vi "user32_SendMessage.vi"(5 "IParam":u32, 7 "wParam":u32, 8 "错误输入（无错误）":errorcluster, 9 "Msg":u32, 10 "hWnd":u32, 11 "路径输入":path) -> (0 "错误输出":errorcluster, 3 "返回值":u32)   [LabVIEW 2017]
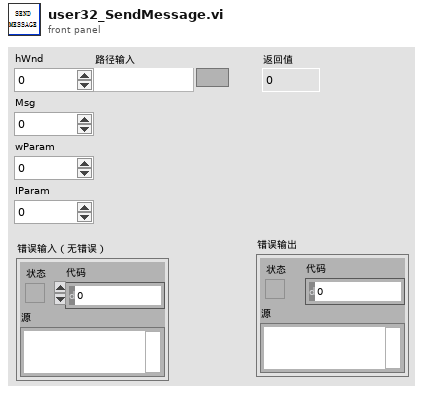
[diagram p1: front panel]
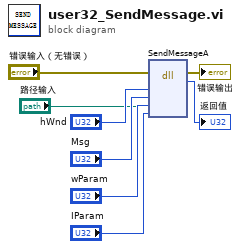
[diagram p0: block diagram]
diagram:
  n1 = dll-call lib="C:/Windows/System32/user32.dll" fn="SendMessageA"(path in="路径输入", error in="错误输入（无错误）", "hWnd"="hWnd", "Msg"="Msg", "wParam"="wParam", "IParam"="IParam") -> (error out=→"错误输出":errorcluster, "返回值"=→"返回值":u32)  [unwired: 5 in, 1 out]
